vi "MRC Ds Comms Get Control Data.vi"(8 "error in (no error)":errorcluster, 11 "data":T1) -> (0 "error out":errorcluster, 3 "data out":T1)   [LabVIEW 2026, in "MrcLib.lvlib"]
doc: "MRC_Status MRC_CALLCONV MRC_DsComms_GetControlData(struct MRC_ControlData* data);"
uses:
  MrcLib.lvlib
  MRC_ControlData.ctl
  MrcLib.dll
  Types/MRC Str64.ctl
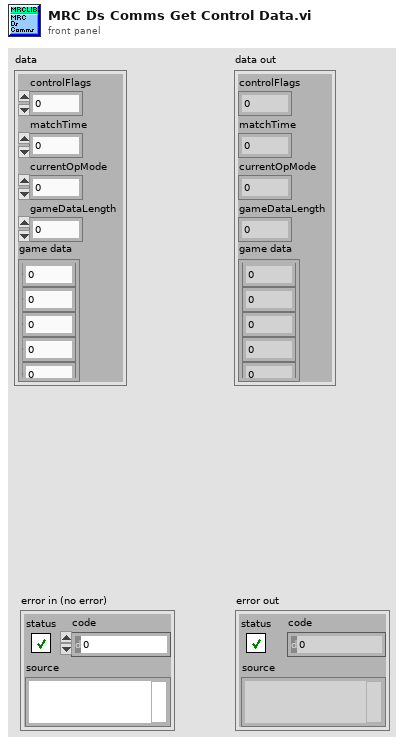
[diagram p1: front panel]
types:
  T1 = typedef "MrcLib.lvlib/MRC_ControlData.ctl" = cluster{"controlFlags":u32, "matchTime":u16, "currentOpMode":u64, "gameDataLength":u8, "game data":T2}
  T2 = typedef "MRC Str64.ctl" = cluster{"[0]":u8, "[1]":u8, "[2]":u8, "[3]":u8, "[4]":u8, "[5]":u8, "[6]":u8, "[7]":u8, "[8]":u8, "[9]":u8, "[10]":u8, "[11]":u8, "[12]":u8, "[13]":u8, "[14]":u8, "[15]":u8, "[16]":u8, "[17]":u8, "[18]":u8, "[19]":u8, "[20]":u8, "[21]":u8, "[22]":u8, "[23]":u8, "[24]":u8, "[25]":u8, "[26]":u8, "[27]":u8, "[28]":u8, "[29]":u8, "[30]":u8, "[31]":u8, "[32]":u8, "[33]":u8, "[34]":u8, "[35]":u8, "[36]":u8, "[37]":u8, "[38]":u8, "[39]":u8, "[40]":u8, "[41]":u8, "[42]":u8, "[43]":u8, "[44]":u8, "[45]":u8, "[46]":u8, "[47]":u8, "[48]":u8, "[49]":u8, "[50]":u8, "[51]":u8, "[52]":u8, "[53]":u8, "[54]":u8, "[55]":u8, "[56]":u8, "[57]":u8, "[58]":u8, "[59]":u8, "[60]":u8, "[61]":u8, "[62]":u8, "[63]":u8}
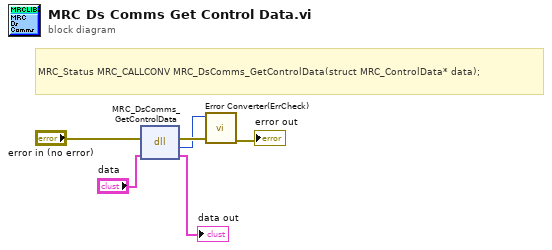
[diagram p0: block diagram]
diagram:
  # "MRC_Status MRC_CALLCONV MRC_DsComms_GetControlData(struct MRC_ControlData* data);"
  n1 = dll-call lib="MrcLib.*" fn="MRC_DsComms_GetControlData"(error in="error in (no error)", "data"="data") -> (error out=w3:errorcluster, "return type"=w1:i32, "data"=→"data out":T1)  [unwired: 2 in, 1 out]
  n2 = call "Error Converter(ErrCheck).vi"("error in (no error)"=w3, "status"=w1) -> ("error out"=→"error out":errorcluster)  [unwired: 9 in]
